vi "onKeyWrite.vi"(7 "Qualified Name":string[](array[string]), 8 "error in (no error)":errorcluster, 9 "Content":T1[](array[typedef]), 10 "Keys":string[](array[string]), 11 "ConfigManager.Text in":refnum<class "ConfigManager.Text.lvclass">) -> (0 "error out":errorcluster, 1 "Content out":T1[](array[typedef]), 2 "Keys out":string[](array[string]), 3 "ConfigManager.Text out":refnum<class "ConfigManager.Text.lvclass">, 5 "Qualified Name out":string[](array[string]))   [LabVIEW 2013, in "CfgManager.Text.lvlib" / "ConfigManager.Text.lvclass"]
uses:
  ConfigManager.Text.lvclass
  Dictionary Payload -- cluster.ctl
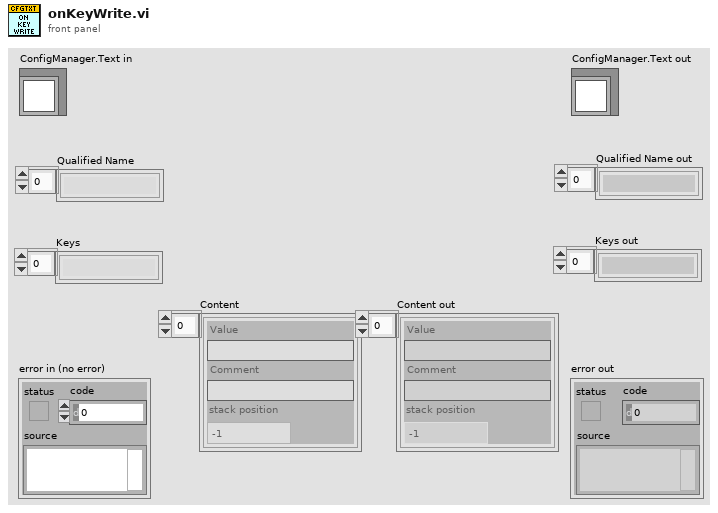
[diagram p1: front panel]
types:
  T1 = typedef "CfgManager.Text.lvlib/ConfigManager.Text.lvclass/Dictionary Payload -- cluster.ctl" = cluster{"Value":string, "Comment":string, "stack position":i32}
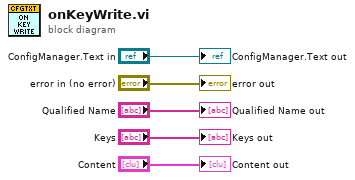
[diagram p0: block diagram]
diagram:
  "error out" <- "error in (no error)"
  "ConfigManager.Text out" <- "ConfigManager.Text in"
  "Keys out" <- "Keys"
  "Qualified Name out" <- "Qualified Name"
  "Content out" <- "Content"
